vi "Persist Config.vi"(8 "error in (no error)":errorcluster, 10 "Root":refnum<class "Config Element.lvclass">, 11 "Config-INI in":refnum<class "Config-INI.lvclass">) -> (0 "error out":errorcluster, 3 "Config-INI out":refnum<class "Config-INI.lvclass">)   [LabVIEW 2020, in "CDM-Config.lvlib" / "Config-INI.lvclass"]
uses:
  Config-INI.lvclass
  C:/dev/lv20CE/lv-cdm/CDM-Config/Config Storage/Config Storage.lvclass
  Config Element/Config Element.lvclass
  Config-INI.lvclass/Config-INI.ctl
  <vilib>/AdvancedString/1D String Array to Delimited String.vi
  <vilib>/Utility/config.llb/Write Key (String).vi
  <vilib>/Utility/config.llb/NI_LVConfig.lvlib
  CDM-Config.lvlib
  Config Storage/Config Storage.lvclass
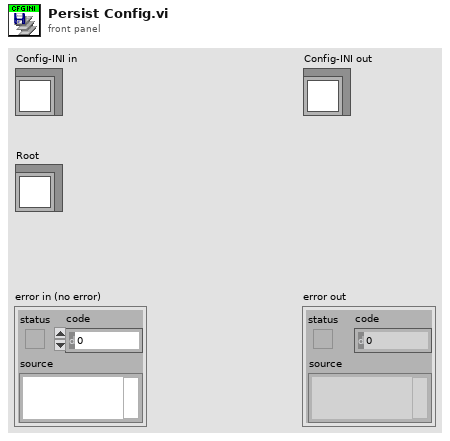
[diagram p1: front panel]
types:
  T1 = typedef "NI_LVConfig.lvlib/Config Data RefNum.ctl" = refnum<k1>
  T2 = typedef "CDM-Config.lvlib/Meta Data.ctl" = cluster{"Name":string, "Value":string}
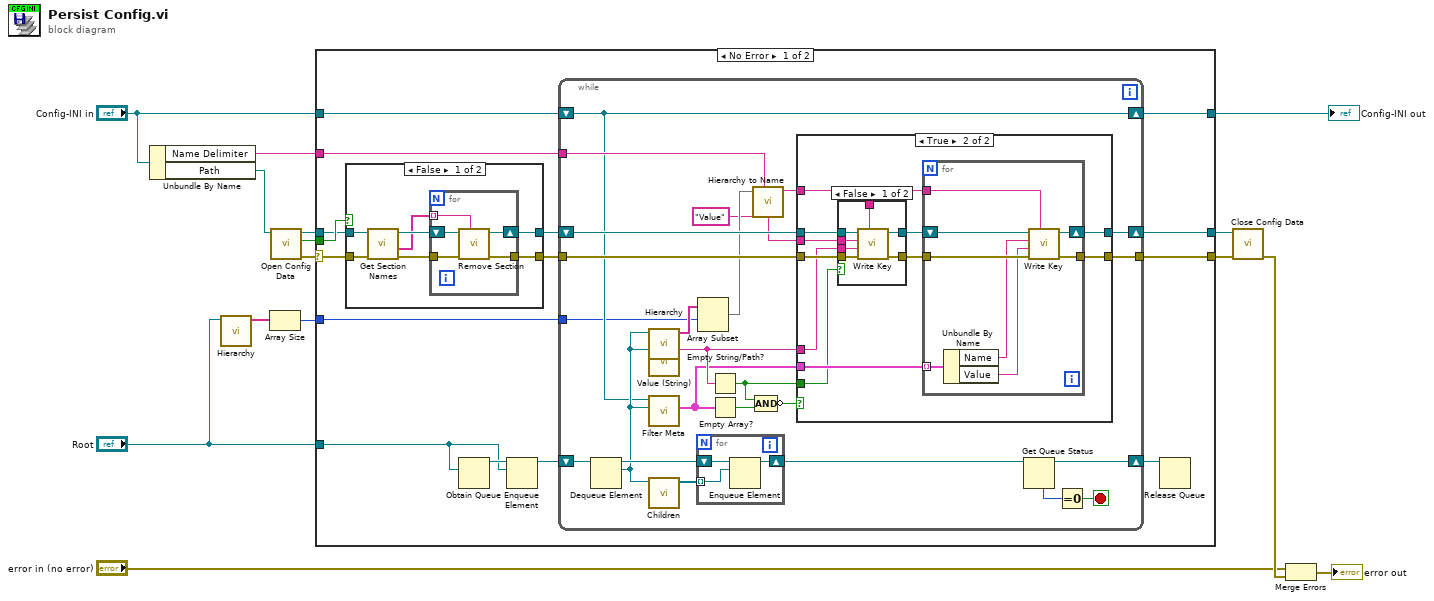
[diagram p0: block diagram]
diagram:
  n1 = Unbundle By Name("Config-INI in") -> ("Name Delimiter"=w6:string, "Path"=w15:path)
  n2 = call "Hierarchy.vi"("Config Element in"="Root") -> ("Hierarchy"=w2:string[])  [unwired: 9 in, 1 out]
  n3 = Array Size(array=w2) -> (size(s)=w3:i32)
  n4 = call <vilib>:"Open Config Data.vi"("configuration file path"=w15) -> ("error out"=w14:errorcluster, "file created?"=w12:bool, "refnum"=w13:T1)  [unwired: 8 in]
  n5 = case shown="No Error" w14 {
    selector: w14 -> [w28 w103]
    tunnel: w13 -> [w29 w104]
    tunnel: "Root" -> [w21 _]
    tunnel: w12 -> [w30 _]
    tunnel: [w25 w104] -> w11
    tunnel: [w24 w103] -> w10
    tunnel: w6 -> [w23 _]
    tunnel: "Config-INI in" -> [w18 w102]
    tunnel: [w17 w102] -> w5
    tunnel: w3 -> [w16 _]
    frame No Error {
      n6 = case shown="False" w30 {
        tunnel: w29 -> [w37 w44]
        tunnel: w28 -> [w36 w43]
        tunnel: [w32 w44] -> w27
        tunnel: [w31 w43] -> w26
        frame False {
          n7 = call <vilib>:"Get Section Names.vi"("error in (no error)"=w36, "refnum"=w37) -> ("error out"=w35:errorcluster, "section names"=w33:string[], "refnum out"=w34:T1)  [unwired: 7 in]
          n8 = for {
            tunnel: w35 -> [w41]
            shift-right: [w40] -> w32
            shift-left: w34 -> [w42]
            tunnel: [w39] -> w31
            tunnel: w33 -> [w38] mode=indexing
            n9 = call <vilib>:"Remove Section.vi"("section"=w38, "error in (no error)"=w41, "refnum"=w42) -> ("error out"=w39:errorcluster, "refnum out"=w40:T1)  [unwired: 6 in, 1 out]
          }
        }
        frame True {
        }
      }
      n10 = Obtain Queue(element data type=w21) -> (queue out=w22:refnum<queue>)  [unwired: 4 in, 2 out]
      n11 = Enqueue Element(queue=w22, element=w21) -> (queue out=w20:refnum<queue>)  [unwired: 2 in, 2 out]
      n12 = while {
        shift-right: [w66] -> w25
        shift-left: w27 -> [w68]
        tunnel: w26 -> [w67]
        tunnel: [w65] -> w24
        tunnel: w23 -> [w63]
        shift-right: [w59] -> w19
        shift-left: w20 -> [w62]
        shift-right: [w46] -> w17
        shift-left: w18 -> [w46]
        tunnel: w16 -> [w45]
        stop <- w58 stop-if-true
        n13 = Dequeue Element(queue=w62) -> (queue out=w61:refnum<queue>, element=w57:refnum<class "Config Element.lvclass">)  [unwired: 2 in, 2 out]
        n14 = call "Hierarchy.vi"("Config Element in"=w57) -> ("Hierarchy"=w55:string[])  [unwired: 9 in, 1 out]
        n15 = call "Value (String).vi"("Config Element in"=w57) -> ("String Value"=w64:string)  [unwired: 9 in, 1 out]
        n16 = call "Filter Meta.vi"("Element"=w57, "Config Storage in"=w46) -> ("Filtered Meta"=w56:T2[])  [unwired: 7 in, 2 out]
        n17 = call "Children.vi"("Config Element in"=w57) -> ("Elements"=w60:refnum<class "Config Element.lvclass">[])  [unwired: 9 in, 1 out]
        n18 = for {
          shift-right: [w69] -> w48
          shift-left: w61 -> [w71]
          tunnel: w60 -> [w70] mode=indexing
          n19 = Enqueue Element(queue=w71, element=w70) -> (queue out=w69:refnum<queue>)  [unwired: 2 in, 2 out]
        }
        n20 = Array Subset(array=w55, index=w45) -> (w54:string[])  [unwired: 1 in]
        n21 = Empty String/Path?(string/path=w64) -> (empty?=w49:bool)
        n22 = Empty Array?(array=w56) -> (empty?=w51:bool)
        n23 = call "Hierarchy to Name.vi"("Delimiter"=w63, "Hierarchy"=w54) -> ("Full Name"=w52:string)  [unwired: 9 in]
        n24 = Compound Arithmetic op=AND(w49, w51) -> (invert w50:bool)
        n25 = case shown="True" w50 {
          tunnel: w68 -> [w73 w84]
          tunnel: w67 -> [w72 w83]
          tunnel: "Value" ("key") -> [_ w82]
          tunnel: [w73 w79] -> w66
          tunnel: [w72 w78] -> w65
          tunnel: w52 -> [_ w77]
          tunnel: w64 -> [_ w76]
          tunnel: w56 -> [_ w75]
          tunnel: w49 -> [_ w74]
          frame False {
          }
          frame True {
            n26 = case shown="False" w74 {
              tunnel: w84 -> [w91 w93]
              tunnel: w83 -> [w90 w92]
              tunnel: w82 -> [w89 _]
              tunnel: [w88 w93] -> w81
              tunnel: [w87 w92] -> w80
              tunnel: w77 -> [w86 _]
              tunnel: w76 -> [w85 _]
              frame False {
                n27 = call-poly <vilib>:"Write Key.vi"("section"=w86, "error in (no error)"=w90, "value"=w85, "key"=w89, "refnum"=w91) -> ("error out"=w87:errorcluster, "refnum out"=w88:T1)  [unwired: 4 in, 1 out]
              }
              frame True {
              }
            }
            n28 = for {
              shift-right: [w95] -> w79
              shift-left: w81 -> [w101]
              tunnel: w80 -> [w100]
              tunnel: w75 -> [w98] mode=indexing
              tunnel: w77 -> [w99]
              tunnel: [w94] -> w78
              n29 = Unbundle By Name(w98) -> ("Name"=w97:string, "Value"=w96:string)
              n30 = call-poly <vilib>:"Write Key.vi"("section"=w99, "error in (no error)"=w100, "value"=w96, "key"=w97, "refnum"=w101) -> ("error out"=w94:errorcluster, "refnum out"=w95:T1)  [unwired: 4 in, 1 out]
            }
          }
        }
        n31 = Get Queue Status(queue=w48) -> (queue out=w59:refnum<queue>, # elements in queue=w47:i32)  [unwired: 2 in, 6 out]
        n32 = Equal To 0?(x=w47) -> (x = 0?=w58:bool)
      }
      n33 = Release Queue(queue=w19) -> ()  [unwired: 2 in, 3 out]
    }
    frame Error {
    }
  }
  "Config-INI out" <- w5
  n34 = call <vilib>:"Close Config Data.vi"("error in (no error)"=w10, "refnum"=w11) -> ("error out"=w9:errorcluster)  [unwired: 8 in, 1 out]
  n35 = Merge Errors("error in (no error)", w9) -> (→"error out":errorcluster)
